vi "Read RT Table.vi"(2 "error in (no error)":errorcluster, 3 "Simulator":bool, 4 "key":string) -> (0 "error out":errorcluster, 1 "Table":dbl[][](array[numeric]))   [LabVIEW 2018]
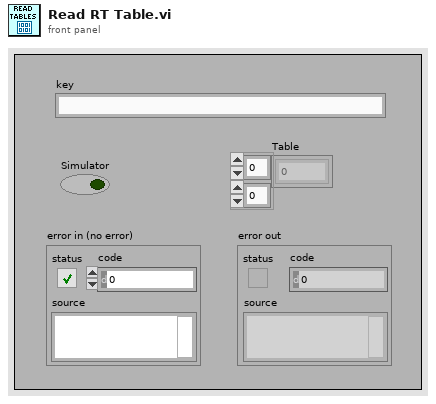
[diagram p1: front panel]
types:
  T1 = enum16{"open", "replace", "create", "open or create", "replace or create", "replace or create with confirmation"}
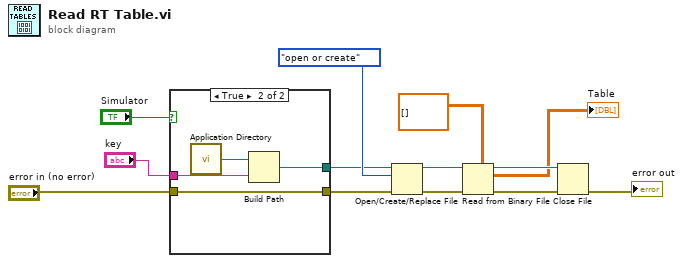
[diagram p0: block diagram]
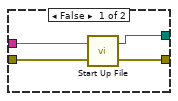
[diagram p2: hidden frame]
diagram:
  n1 = case shown="True" "Simulator" {
    tunnel: "error in (no error)" -> [w15 w19]
    tunnel: [w17 w19] -> w5
    tunnel: [w16 w20] -> w4
    tunnel: "key" -> [w14 w18]
    frame False {
      n2 = call "Start Up File.vi"("error in (no error)"=w15, "FileName"=w14) -> ("error out"=w17:errorcluster, "FilePath"=w16:path)
    }
    frame True {
      n3 = call <vilib>:"Application Directory.vi"() -> ("Application Directory"=w21:path)
      n4 = Build Path(base path=w21, name or relative path=w18) -> (appended path=w20:path)
    }
  }
  n5 = Open/Create/Replace File(file path (use dialog)=w4, error in=w5, operation (0:open)=T1."open or create") -> (refnum out=w10:refnum<file>, error out=w11:errorcluster)  [unwired: 3 in, 1 out]
  n6 = Read from Binary File(5:dbl[][] [], 8:w11, 11:w10) -> (0:w13:errorcluster, 2:→"Table":dbl[][], 3:w12:refnum<file>)  [unwired: 4 out]
  n7 = Close File(refnum=w12, error in=w13) -> (error out=→"error out":errorcluster)  [unwired: 1 out]
